vi "strain-data-buffer2.vi"(7 "cmd":enum16{"ini", "add", "read"}(ring), 8 "wf 4":waveform(dbl), 9 "wf 3":waveform(dbl), 10 "wf 2":waveform(dbl), 11 "wf 1":waveform(dbl)) -> (1 "array index":i32, 2 "wf sup":waveform(dbl) caption="x+y", 3 "wf array":waveform(dbl)[](array[waveform]))   [LabVIEW 2013]
uses:
  ctl/strain_wf_ctl.ctl
  <vilib>/Waveform/WDTOps.llb/WDT Append Waveforms DBL.vi
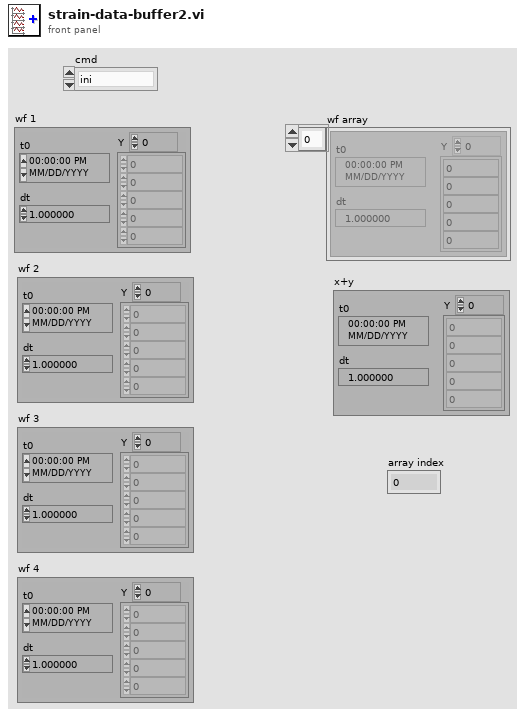
[diagram p1: front panel]
types:
  T1 = typedef "strain_wf_ctl.ctl" = waveform(dbl)
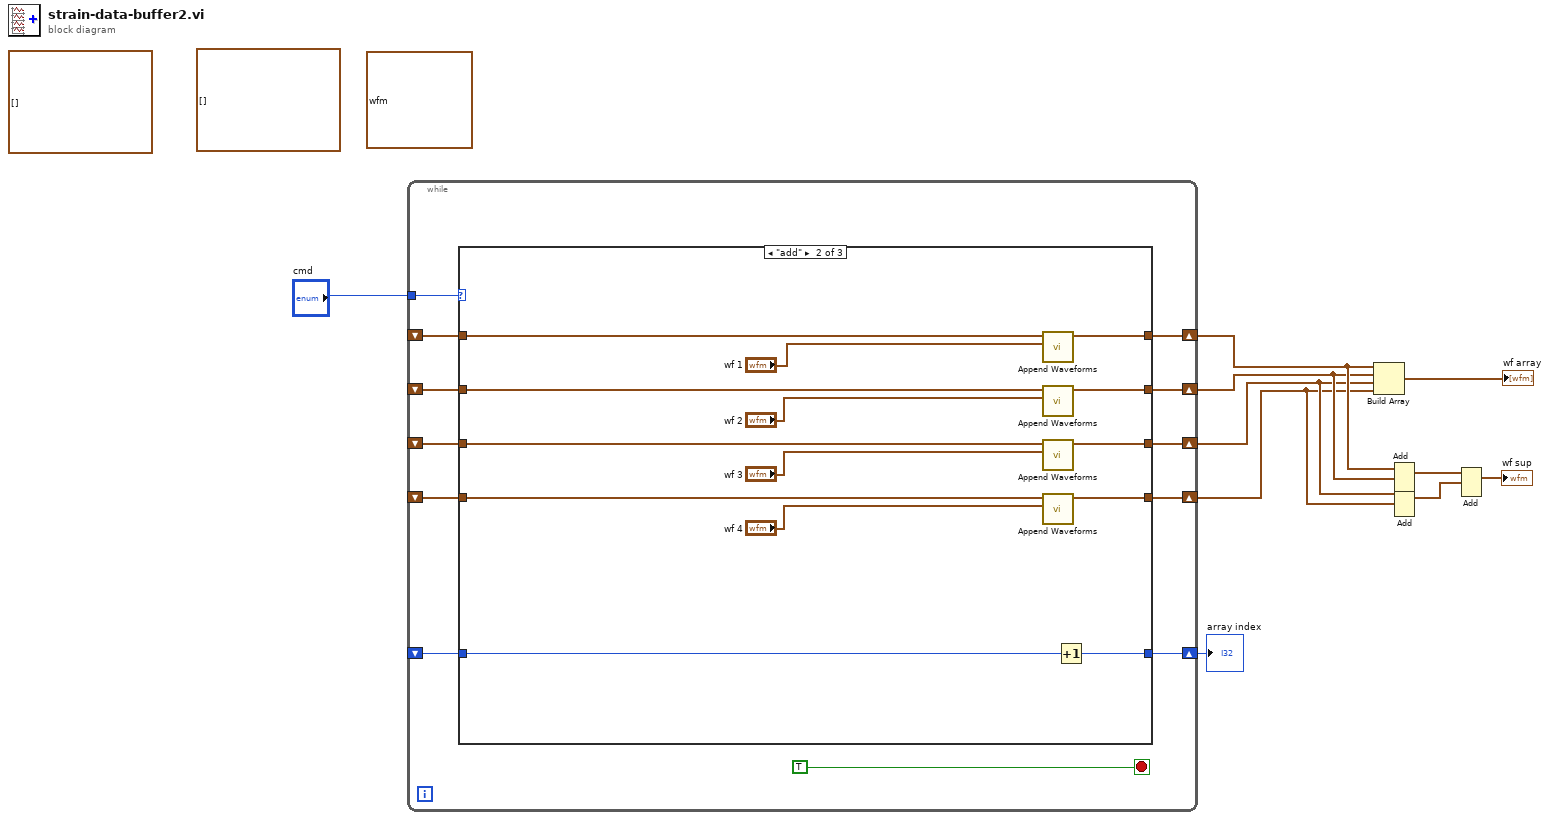
[diagram p0: block diagram]
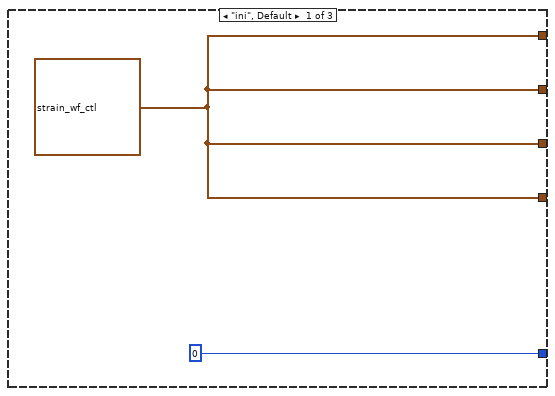
[diagram p2: hidden frame]
diagram:
  (unwired) waveform(dbl)[][] [] ("히스토리 데이터")
  (unwired) waveform(dbl) {"t0"=timestamp(0 s since 1904-01-01), "dt"=1.0, "Y"=[]}
  (unwired) waveform(dbl)[] [] ("History Data")
  n1 = while {
    tunnel: "cmd" -> [w21]
    shift-right: [w20] -> w9
    shift-left: _ -> [w19]
    shift-right: [w18] -> w7
    shift-left: _ -> [w11]
    shift-right: [w15] -> w6
    shift-left: _ -> [w12]
    shift-right: [w16] -> w5
    shift-left: _ -> [w13]
    shift-right: [w17] -> w4
    shift-left: _ -> [w14]
    stop <- TRUE stop-if-true
    n2 = case shown="\"add\"" w21 {
      tunnel: [0 ("array index") w38 w39] -> w20
      tunnel: w19 -> [_ w37 w39]
      tunnel: [w23 w35 w40] -> w18
      tunnel: [w23 w33 w43] -> w17
      tunnel: [w23 w32 w42] -> w16
      tunnel: [w23 w31 w41] -> w15
      tunnel: w14 -> [_ w26 w43]
      tunnel: w13 -> [_ w28 w42]
      tunnel: w12 -> [_ w30 w41]
      tunnel: w11 -> [_ w36 w40]
      frame "ini", Default {
        w23 = T1 {"t0"=timestamp(0 s since 1904-01-01), "dt"=0.00062, "Y"=[]} ("Waveform")
      }
      frame "add" {
        n3 = call-poly <vilib>:"Append Waveforms.vi"("waveform B"="wf 1", "waveform A"=w36) -> ("waveform out"=w35:waveform(dbl))  [unwired: 8 in, 1 out]
        n4 = call-poly <vilib>:"Append Waveforms.vi"("waveform B"="wf 2", "waveform A"=w30) -> ("waveform out"=w31:waveform(dbl))  [unwired: 8 in, 1 out]
        n5 = call-poly <vilib>:"Append Waveforms.vi"("waveform B"="wf 3", "waveform A"=w28) -> ("waveform out"=w32:waveform(dbl))  [unwired: 8 in, 1 out]
        n6 = call-poly <vilib>:"Append Waveforms.vi"("waveform B"="wf 4", "waveform A"=w26) -> ("waveform out"=w33:waveform(dbl))  [unwired: 8 in, 1 out]
        n7 = Increment(x=w37) -> (x+1=w38:i32)
      }
      frame "read" {
      }
    }
  }
  "array index" <- w9
  n8 = Build Array(w7, w6, w5, w4) -> (→"wf array":T1[])
  n9 = Add(1:w6, 2:w7) -> (0:w2:T1)  [unwired: 1 in, 1 out]
  n10 = Add(1:w4, 2:w5) -> (0:w3:T1)  [unwired: 1 in, 1 out]
  n11 = Add(1:w3, 2:w2) -> (0:→"wf sup":T1)  [unwired: 1 in, 1 out]
